vi "PH_gentec_Powermeter.set Statistics Config.vi"(0 "i ref in":refnum<vi>, 2 "VISA resource in":refnum<visa-resource-name>, 4 "Device error in":errorcluster, 5 "error in":errorcluster) -> (14 "i ref out":refnum<vi>, 15 "Timeout":bool, 16 "VISA resource out":refnum<visa-resource-name>, 17 "Error Messages":string, 18 "Device error out":errorcluster, 19 "error out":errorcluster)   [LabVIEW 2014, in "PH_gentec_Powermeter.lvlib"]
doc: "This VI sets the statistics configuration of the powermeter. Then the value queried from the powermeter is set to own attributes and the GUI element."
uses:
  PH_gentec_Powermeter.lvlib
  instr.lib/gentec-SOLO-PE/gentec-SOLO-PE - Driver.lvlib
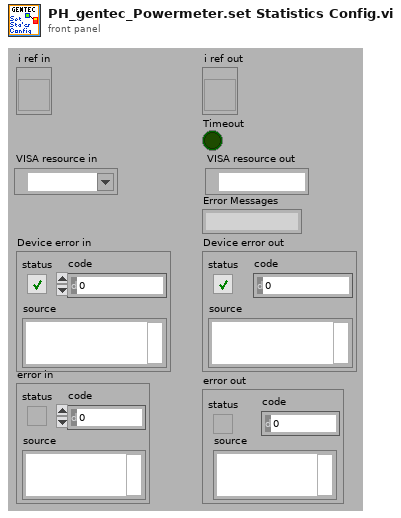
[diagram p1: front panel]
types:
  T1 = typedef "PH_gentec_Powermeter.lvlib/PH_gentec_Powermeter.i attribute.ctl" = cluster{"GUI References":cluster{"delete":refnum<vi>, "start stop Statistics":refnum<vi>, "Statistic Data":refnum<vi>, "Configuration Values":refnum<vi>, "Set Zero":refnum<vi>, "Data Sampling Settings":refnum<vi>, "Wanted Sets":refnum<vi>, "Current Sets":refnum<vi>}, "Start Stop Statistics":bool, "Wanted Sets":T2, "Current Sets":T2}
  T2 = typedef "PH_gentec_Powermeter.lvlib/PH_gentec_Powermeter.Sets.ctl" = cluster{"Data Sampling Settings":T3, "Set Zero":bool}
  T3 = typedef "gentec-SOLO-PE - Driver.lvlib/gentec-SOLO-PE.Data Sampling Settings.ctl" = cluster{"Sample Rate":u32, "Sample Rate Unit":u32, "Sample Period":u32, "Sample Period Unit":u32, "Total Duration":u32, "Total Duration Unit":u32, "Time Stamp":u32}
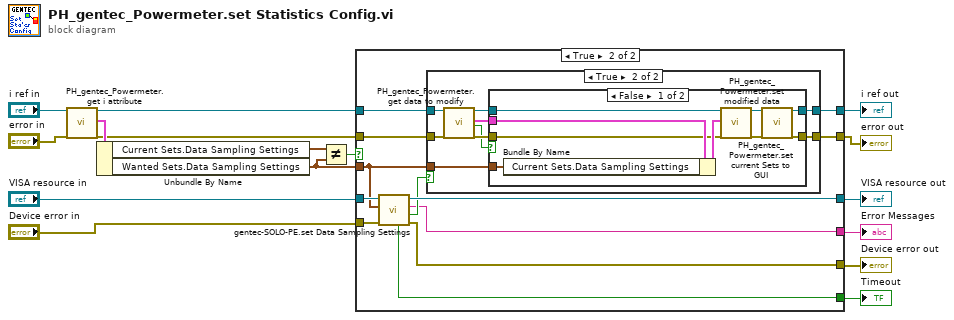
[diagram p0: block diagram]
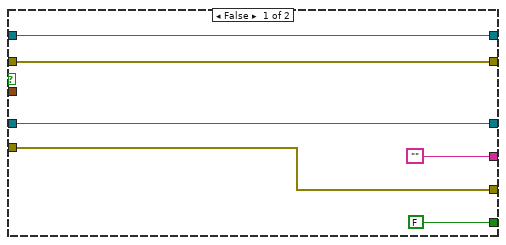
[diagram p2: hidden frame]
diagram:
  n1 = call "PH_gentec_Powermeter.get i attribute.vi"("i ref in"="i ref in", "error in (no error)"="error in") -> ("i ref out"=w8:refnum<vi>, "i attribute"=w12:T1, "error out"=w7:errorcluster)  [unwired: 15 in]
  n2 = Unbundle By Name(w12) -> ("Current Sets.Data Sampling Settings"=w11:T3, "Wanted Sets.Data Sampling Settings"=w10:T3)
  n3 = Not Equal?(x=w11, y=w10) -> (x != y?=w5:bool)
  n4 = case shown="True" w5 {
    tunnel: [w22 w34] -> w16
    tunnel: [w21 w33] -> w14
    tunnel: w10 -> [_ w26]
    tunnel: "VISA resource in" -> [w20 w32]
    tunnel: w8 -> [w22 w31]
    tunnel: w7 -> [w21 w30]
    tunnel: [w20 w28] -> w6
    tunnel: [w19 w27] -> w4
    tunnel: "Device error in" -> [w19 w29]
    tunnel: [FALSE ("Timeout") w24] -> w1
    tunnel: ["" w23] -> w2
    frame False {
    }
    frame True {
      n5 = call "gentec-SOLO-PE.set Data Sampling Settings.vi"("error in (no error)"=w29, "Data Samling Settings"=w26, "VISA Refnum in"=w32) -> ("error out"=w27:errorcluster, "Acknoledged?"=w25:bool, "Error"=w23:string, "VISA Refnum out"=w28:refnum<visa-resource-name>, "Timeout"=w24:bool)  [unwired: 4 in]
      n6 = case shown="True" w25 {
        tunnel: [w36 w41] -> w34
        tunnel: [w35 w40] -> w33
        tunnel: w31 -> [w36 w39]
        tunnel: w30 -> [w35 w38]
        tunnel: w26 -> [_ w37]
        frame False {
        }
        frame True {
          n7 = call "PH_gentec_Powermeter.get data to modify.vi"("i ref in"=w39, "error in (no error)"=w38) -> ("i ref out"=w45:refnum<vi>, "i attribute"=w44:T1, "timed out"=w42:bool, "error out"=w43:errorcluster)  [unwired: 14 in]
          n8 = case shown="False" w42 {
            tunnel: w43 -> [w50 w55]
            tunnel: w45 -> [w53 w56]
            tunnel: [w47 w56] -> w41
            tunnel: [w49 w55] -> w40
            tunnel: w44 -> [w52 _]
            tunnel: w37 -> [w46 _]
            frame False {
              n9 = Bundle By Name(cluster=w52, "Current Sets.Data Sampling Settings"=w46) -> (w51:T1)
              n10 = call "PH_gentec_Powermeter.set modified data.vi"("i ref in"=w53, "i attribute"=w51, "error in (no error)"=w50) -> ("i ref out"=w48:refnum<vi>, "error out"=w54:errorcluster)  [unwired: 15 in]
              n11 = call "PH_gentec_Powermeter.set current Sets to GUI.vi"("i ref in"=w48, "error in"=w54) -> ("i ref out"=w47:refnum<vi>, "error out"=w49:errorcluster)  [unwired: 16 in]
            }
            frame True {
            }
          }
        }
      }
    }
  }
  "error out" <- w14
  "i ref out" <- w16
  "VISA resource out" <- w6
  "Device error out" <- w4
  "Error Messages" <- w2
  "Timeout" <- w1
